vi "(SubVI) Calculate ACF .vi"(4 "ACF length":i32=300, 5 "dt":dbl, 6 "Data":dbl[](array[numeric])) -> (1 "ACF":dbl[](array[numeric]), 2 "x or t":dbl[](array[numeric]))   [LabVIEW 2014]
uses:
  <vilib>/Analysis/2dsp.llb/1D Auto Correlation (DBL).vi
  <vilib>/Analysis/NI_AALPro.lvlib
panel:
  out "size(s)":i32
  out "Waveform Graph":dbl[](graph)
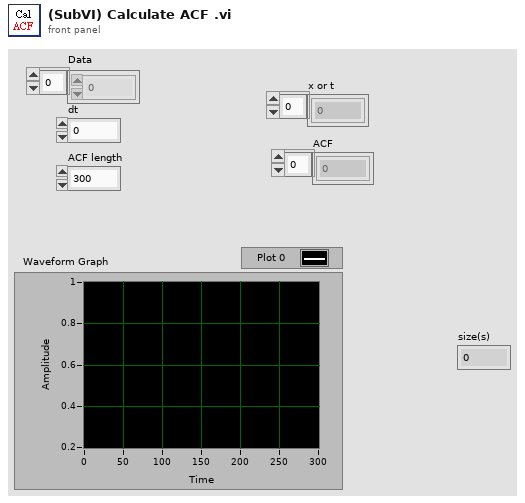
[diagram p1: front panel]
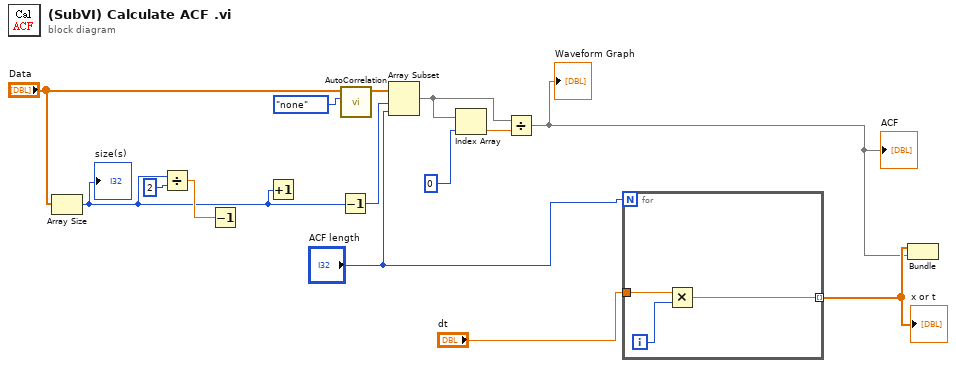
[diagram p0: block diagram]
diagram:
  n1 = Array Size(array="Data") -> (size(s)=w11:i32)
  "size(s)" <- w11
  n2 = Divide(x=w11, y=2) -> (x/y=w12:dbl)
  n3 = Decrement(x=w12) -> ()  [unwired: 1 out]
  n4 = Increment(x=w11) -> ()  [unwired: 1 out]
  n5 = Decrement(x=w11) -> (x-1=w8:i32)
  n6 = call-poly <vilib>:"AutoCorrelation.vi"("normalization"=enum32{"none", "unbiased", "biased"}."none", "X"="Data") -> ("Rxx"=w9:dbl[])  [unwired: 8 in, 1 out]
  n7 = Array Subset(array=w9, index=w8, length="ACF length") -> (w5:dbl[])
  n8 = Index Array(array=w5, index=0) -> (element=w6:dbl)
  n9 = Divide(x=w5, y=w6) -> (x/y=w1:dbl[])
  "Waveform Graph" <- w1
  "ACF" <- w1
  n10 = for {
    N: "ACF length" -> [_]
    tunnel: "dt" -> [w16]
    tunnel: [w15] -> w2 mode=indexing
    i -> [w17]
    n11 = Multiply(x=w16, y=w17) -> (x*y=w15:dbl)
  }
  "x or t" <- w2
  n12 = Bundle(w2, w1) -> ()  [unwired: 1 in, 1 out]
